vi "Reset Dev.vi"(8 "error in (no error)":errorcluster, 11 "hdwf":i32) -> (0 "error out":errorcluster, 3 "function return":i32)   [LabVIEW 2012, in "AnalogDiscSDKLv.lvlib"]
doc: "extern \"C\" __declspec(dllexport) int Reset_DevLv(HDWF hdwf);"
uses:
  <instrlib>/AnalogDiscSDKLv/AnalogDiscSDKLv.lvlib
  <instrlib>/AnalogDiscSDKLv/AnalogDiscSDKLv.dll
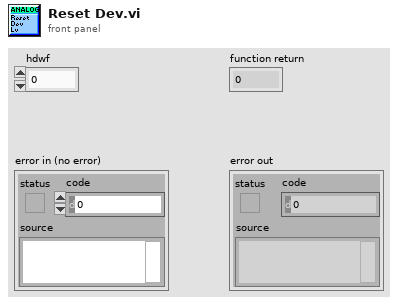
[diagram p1: front panel]
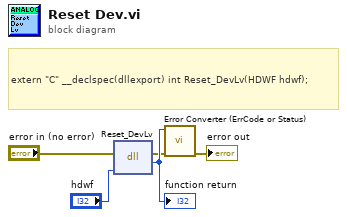
[diagram p0: block diagram]
diagram:
  # "extern \"C\" __declspec(dllexport) int Reset_DevLv(HDWF hdwf);"
  n1 = dll-call lib="C:/Program Files (x86)/National Instruments/LabVIEW 2012/instr.lib/AnalogDiscSDKLv/AnalogDiscSDKLv.*" fn="Reset_DevLv"(error in="error in (no error)", "hdwf"="hdwf") -> (error out=w2:errorcluster, w5:i32)  [unwired: 3 in, 1 out]
  "function return" <- w5
  n2 = call <instrlib>:"Error Converter (ErrCode or Status).vi"("error in (no error)"=w2, "error code"=w5) -> ("error out"=→"error out":errorcluster)  [unwired: 9 in]
